vi "Conversion tension température.vi"(11 "Tension In":dbl[](array[numeric])) -> (3 "Température Out":dbl[](array[numeric]))   [LabVIEW 2018]
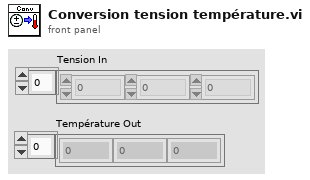
[diagram p1: front panel]
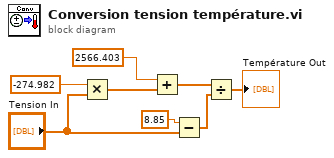
[diagram p0: block diagram]
diagram:
  n1 = Multiply(x=-274.982, y="Tension In") -> (x*y=w2:dbl[])
  n2 = Add(x=2566.403, y=w2) -> (x+y=w1:dbl[])
  n3 = Subtract(x=8.85, y="Tension In") -> (x-y=w6:dbl[])
  n4 = Divide(x=w1, y=w6) -> (x/y=→"Température Out":dbl[])
